vi "Populate Menu Items.vi"(8 "error in (no error)":errorcluster, 11 "InsertionPalettePanel in":refnum<class "InsertionPalettePanel.lvclass">) -> (0 "error out":errorcluster, 3 "InsertionPalettePanel out":refnum<class "InsertionPalettePanel.lvclass">)   [LabVIEW 2020, in "TSnax UI.lvlib" / "InsertionPalettePanel.lvclass"]
uses:
  InsertionPalettePanel.lvclass
  InsertionPalettePanel.lvclass/InsertionPalettePanel.ctl
  StepTypeMenuItem/StepTypeMenuItem.lvclass
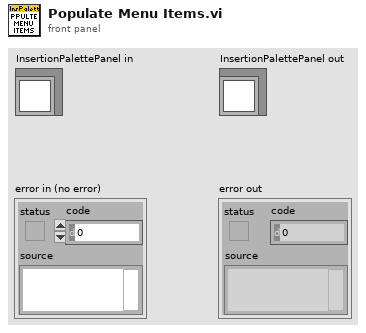
[diagram p1: front panel]
types:
  T1 = typedef "TSnax UI.lvlib/InsertionPalettePanel.lvclass/Ref Data.ctl" = cluster{"Menu Items":map{string, refnum<class "StepTypeMenuItem.lvclass">}}
  T2 = map{string, refnum<class "StepTypeMenuItem.lvclass">}
  T3 = cluster{"index of element":i32, "Menu Item":refnum<class "StepTypeMenuItem.lvclass">}
  T4 = cluster{"index of element":i32, "Menu Item":refnum<class "StepTypeMenuItem.lvclass">}[]
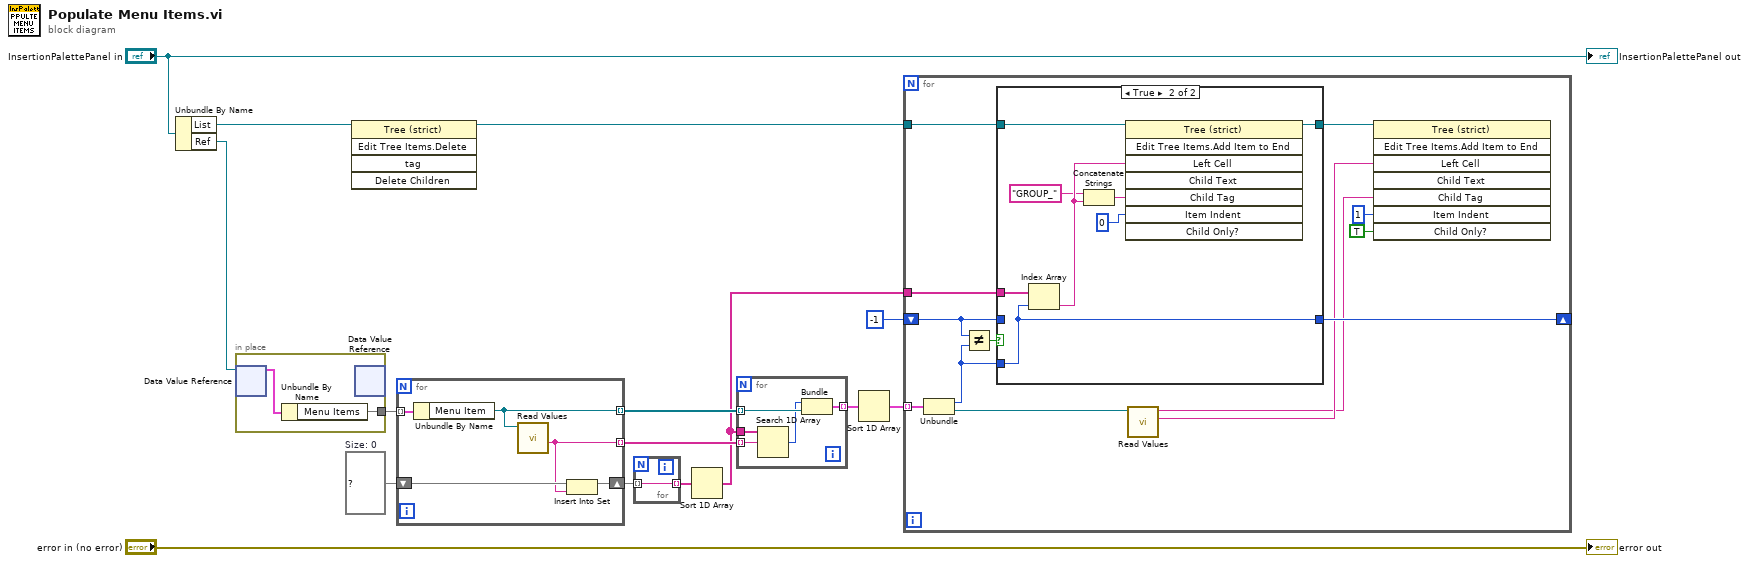
[diagram p0: block diagram]
diagram:
  w11 = set{string} {}  # Size: 0
  n1 = Unbundle By Name("InsertionPalettePanel in") -> ("List"=w3:refnum<vi>, "Ref"=w13:refnum<data-value>)
  n2 = in-place {
    in-place-border: [w16] -> w12
    n3 = in-place-dvr #1(w13) -> (w17:T1)  [unwired: 1 out]
    n4 = Unbundle By Name(w17) -> ("Menu Items"=w16:T2)
    n5 = in-place-dvr #1() -> ()  [unwired: 1 in, 2 out]
  }
  n6 = invoke class="Tree (strict)" method="Edit Tree Items.Delete"(reference=w3) -> (reference out=w2:refnum<vi>)  [unwired: 4 in, 4 out]
  n7 = for {
    tunnel: w12 -> [w22] mode=indexing
    shift-right: [w20] -> w10
    shift-left: w11 -> [w21]
    tunnel: [w19] -> w8 mode=indexing
    tunnel: [w18] -> w7 mode=indexing
    n8 = Unbundle By Name(w22) -> ("Menu Item"=w19:refnum<class "StepTypeMenuItem.lvclass">)
    n9 = call "Read Values.vi"("StepTypeMenuItem in"=w19) -> ("Group"=w18:string)  [unwired: 8 in, 2 out]
    n10 = Insert Into Set(10:w18, 11:w21) -> (3:w20:set{string})  [unwired: 1 out]
  }
  n11 = for {
    tunnel: w10 -> [w23] mode=indexing
    tunnel: [w23] -> w9 mode=indexing
  }
  n12 = Sort 1D Array(array=w9) -> (sorted array=w1:string[])
  n13 = for {
    tunnel: w8 -> [w26] mode=indexing
    tunnel: w7 -> [w27] mode=indexing
    tunnel: w1 -> [w28]
    tunnel: [w24] -> w6 mode=indexing
    n14 = Search 1D Array(1D array=w28, element=w27) -> (index of element=w25:i32)  [unwired: 1 in]
    n15 = Bundle("index of element"=w25, "Menu Item"=w26) -> (w24:T3)  [unwired: 1 in]
  }
  n16 = Sort 1D Array(array=w6) -> (sorted array=w5:T4)
  n17 = for {
    tunnel: w5 -> [w41] mode=indexing
    tunnel: w2 -> [w35]
    shift-right: [w36] -> _
    shift-left: -1 -> [w38]
    tunnel: w1 -> [w40]
    n18 = Unbundle(w41) -> ("index of element"=w37:i32, "Menu Item"=w34:refnum<class "StepTypeMenuItem.lvclass">)
    n19 = Not Equal?(x=w38, y=w37) -> (x != y?=w39:bool)
    n20 = case shown="True" w39 {
      tunnel: w40 -> [_ w49]
      tunnel: w38 -> [w42 _]
      tunnel: w37 -> [_ w48]
      tunnel: [w42 w48] -> w36
      tunnel: w35 -> [w43 w51]
      tunnel: [w43 w44] -> w33
      frame False {
      }
      frame True {
        n21 = Index Array(array=w49, index=w48) -> (element=w46:string)
        n22 = Concatenate Strings("GROUP_" ("string"), w46) -> (w47:string)
        n23 = invoke class="Tree (strict)" method="Edit Tree Items.Add Item to End"(reference=w51, "Left Cell"=w46, "Child Tag"=w47, "Item Indent"=0 ("New Item Indentation")) -> (reference out=w44:refnum<vi>)  [unwired: 4 in, 7 out]
      }
    }
    n24 = call "Read Values.vi"("StepTypeMenuItem in"=w34) -> ("Display Name"=w32:string, "Step Type"=w31:string)  [unwired: 8 in, 1 out]
    n25 = invoke class="Tree (strict)" method="Edit Tree Items.Add Item to End"(reference=w33, "Left Cell"=w32, "Child Tag"=w31, "Item Indent"=1 ("New Item Indentation"), "Child Only?"=TRUE) -> ()  [unwired: 3 in, 8 out]
  }
  "error out" <- "error in (no error)"
  "InsertionPalettePanel out" <- "InsertionPalettePanel in"
